vi "DAQmx_ControlLoop.vi"(8 "error in":errorcluster, 10 "DAQmx Task Name":refnum<k21>="MyVoltageTask_0", 11 "queue out":refnum<queue>) -> (0 "error out":errorcluster)   [LabVIEW 2013]
uses:
  DAQmx_Status.ctl
  <vilib>/Utility/error.llb/DialogType.ctl
  <vilib>/DAQmx/read.llb/DAQmx Read.vi
  <vilib>/DAQmx/read.llb/DAQmx Read (Analog 2D DBL NChan NSamp).vi
  <vilib>/Analysis/baseanly.llb/Mean (DBL).vi
  <vilib>/DAQmx/miscellaneous.llb/DAQmx Fill In Error Info.vi
  ControlDef/MiscParams.vi
  <vilib>/Analysis/NI_AALBase.lvlib
  <userlib>/Utility/ErrorLog_lib.lvlib
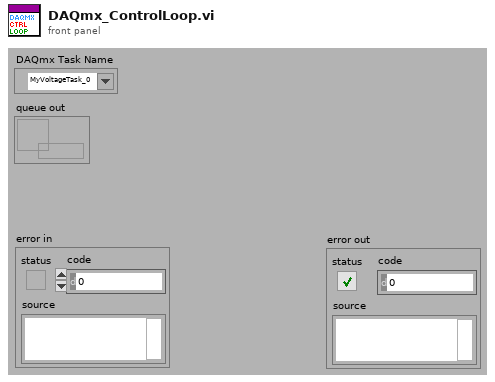
[diagram p1: front panel]
types:
  T1 = typedef "DAQmx_Status.ctl" = cluster{"State":enum16{"Initialize", "Idle", "Update", "Close", "Quit"}, "Para.":variant}
  T2 = enum16{"Initialize", "Idle", "Update", "Close", "Quit"}
  T3 = typedef "DialogType.ctl" = u16
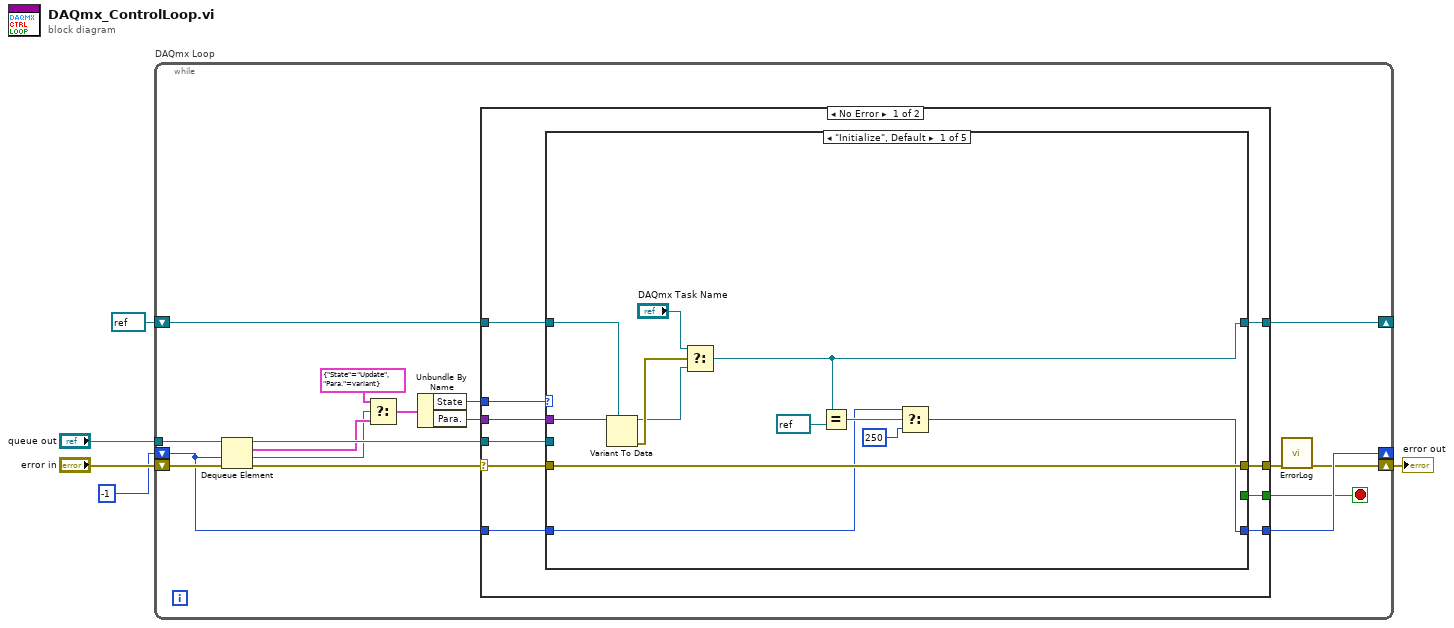
[diagram p0: block diagram]
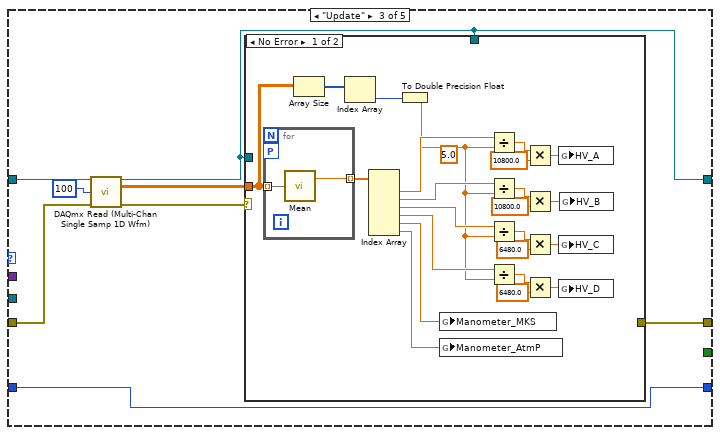
[diagram p3: hidden frame]
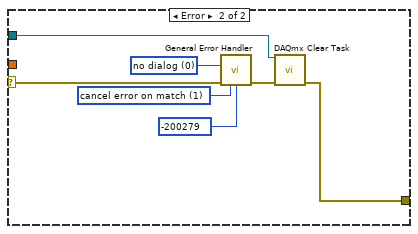
[diagram p4: hidden frame]
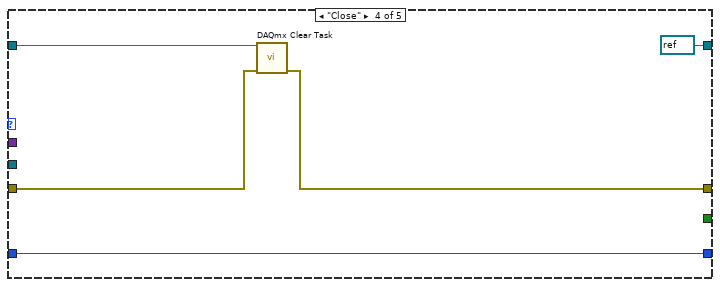
[diagram p5: hidden frame]
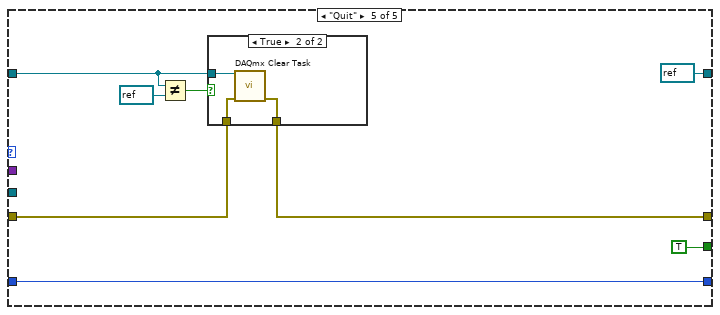
[diagram p6: hidden frame]
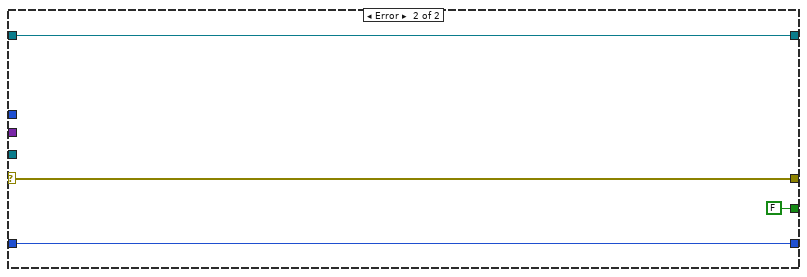
[diagram p8: hidden frame]
diagram:
  n1 = while "DAQmx Loop" {
    tunnel: "queue out" -> [w22]
    shift-right: [w7] -> w2
    shift-left: "error in" -> [w13]
    shift-right: [w11] -> _
    shift-left: refnum<k21> refnum ("DAQmx Task Name") -> [w10]
    shift-right: [w8] -> _
    shift-left: -1 -> [w9]
    stop <- w6 stop-if-true
    n2 = Dequeue Element(queue=w22, timeout in ms (-1)=w9, error in (no error)=w13) -> (queue out=w20:refnum<queue>, element=w17:T1, timed out?=w15:bool, error out=w19:errorcluster)
    n3 = Select(t=T1 {"State"=enum."Update", "Para."=variant}, s=w15, f=w17) -> (s? t:f=w18:T1)
    n4 = Unbundle By Name(w18) -> ("State"=w16:T2, "Para."=w21:variant)
    n5 = case shown="No Error" w19 {
      selector: w19 -> [w29 w108]
      tunnel: w16 -> [w32 _]
      tunnel: w21 -> [w24 _]
      tunnel: w20 -> [w27 _]
      tunnel: [w28 w108] -> w12
      tunnel: [w31 w107] -> w11
      tunnel: w10 -> [w30 w107]
      tunnel: w9 -> [w26 w106]
      tunnel: [w25 w106] -> w8
      tunnel: [w23 FALSE] -> w6
      frame No Error {
        n6 = case shown="\"Initialize\", Default" w32 {
          tunnel: [w37 w47 w49 refnum<k21> refnum ("DAQmx Task Name") refnum<k21> refnum ("DAQmx Task Name")] -> w31
          tunnel: w30 -> [w42 w47 w55 w92 w95]
          tunnel: w29 -> [w44 w46 w54 w91 w99]
          tunnel: [w44 w46 w50 w90 w98] -> w28
          tunnel: w27 -> [_ _ _ _ _]
          tunnel: w26 -> [w34 w45 w48 w88 w94]
          tunnel: [w35 w45 w48 w88 w94] -> w25
          tunnel: w24 -> [w43 _ _ _ _]
          tunnel: [_ _ _ _ TRUE] -> w23
          frame "Initialize", Default {
            n7 = Variant To Data(type=w42, Variant=w43) -> (data=w40:refnum<k21>, error out=w41:errorcluster)  [unwired: 1 in]
            n8 = Select(t="DAQmx Task Name", s=w41, f=w40) -> (s? t:f=w37:refnum<k21>)
            n9 = Equal?(x=w37, y=refnum<k21> refnum ("DAQmx Task Name")) -> (x = y?=w36:bool)
            n10 = Select(t=w34, s=w36, f=250) -> (s? t:f=w35:i32)
          }
          frame "Idle" {
          }
          frame "Update" {
            n11 = call-poly "DAQmx Read (Multi-Chan Single Samp 1D Wfm).vi"("task/channels in"=w55, "number of samples per channel"=100, "error in"=w54) -> ("task out"=w49:refnum<k21>, "data"=w52:dbl[][], "error out"=w51:errorcluster)  [unwired: 10 in]
            n12 = case shown="No Error" w51 {
              selector: w51 -> [_ w87]
              tunnel: w52 -> [w59 _]
              tunnel: [_ w83] -> w50
              tunnel: w49 -> [_ w82]
              tunnel: w49 -> [_ _]
              frame No Error {
                (unwired) 5.0 ("y")
                n13 = for {
                  tunnel: w59 -> [w80] mode=indexing
                  tunnel: [w79] -> w66 mode=indexing
                  workers-P: _ -> [_]
                  n14 = call-poly <vilib>:"Mean.vi"("X"=w80) -> ("mean"=w79:dbl)  [unwired: 1 out]
                }
                n15 = Array Size(array=w59) -> (size(s)=w58:i32[])
                n16 = Index Array(array=w58) -> (element=w57:i32)  [unwired: 1 in]
                n17 = Index Array(array=w66) -> (element #1=w65:dbl, element #2=w64:dbl, element #3=w63:dbl, element #4=w62:dbl, element #5=w61:dbl, element #6=w60:dbl)  [unwired: 6 in]
                n18 = To Double Precision Float(number=w57) -> (double precision float=w56:dbl)
                n19 = global write "MiscParams.vi" "Manometer_MKS"(w61) -> ()
                n20 = global write "MiscParams.vi" "Manometer_AtmP"(w60) -> ()
                n21 = Divide(x=w65, y=w56) -> (x/y=w78:dbl)
                n22 = Divide(x=w64, y=w56) -> (x/y=w75:dbl)
                n23 = Divide(x=w63, y=w56) -> (x/y=w71:dbl)
                n24 = Divide(x=w62, y=w56) -> (x/y=w72:dbl)
                n25 = Multiply(x=w78, y=10800.0) -> (x*y=w70:dbl)
                n26 = Multiply(x=w75, y=10800.0) -> (x*y=w69:dbl)
                n27 = Multiply(x=w71, y=6480.0) -> (x*y=w68:dbl)
                n28 = Multiply(x=w72, y=6480.0) -> (x*y=w67:dbl)
                n29 = global write "MiscParams.vi" "HV_A"(w70) -> ()
                n30 = global write "MiscParams.vi" "HV_C"(w68) -> ()
                n31 = global write "MiscParams.vi" "HV_D"(w67) -> ()
                n32 = global write "MiscParams.vi" "HV_B"(w69) -> ()
              }
              frame Error {
                w81 = T3 0 items=["no dialog", "OK message", "continue or stop message", "OK message + warnings", "continue/stop + warnings"] ("type of dialog (OK msg:1)")
                w86 = 1 items=["no exception", "cancel error on match", "set error on match"] ("[exception action] (none:0)")
                n33 = call <vilib>:"General Error Handler.vi"("type of dialog (OK msg:1)"=w81, "error in (no error)"=w87, "[exception action] (none:0)"=w86, "[exception code]"=-200279) -> ("error out"=w84:errorcluster)  [unwired: 7 in, 4 out]
                n34 = call <vilib>:"DAQmx Clear Task.vi"("task in"=w82, "error in"=w84) -> ("error out"=w83:errorcluster)  [unwired: 13 in]
              }
            }
          }
          frame "Close" {
            n35 = call <vilib>:"DAQmx Clear Task.vi"("task in"=w92, "error in"=w91) -> ("error out"=w90:errorcluster)  [unwired: 13 in]
          }
          frame "Quit" {
            n36 = Not Equal?(x=w95, y=refnum<k21> refnum ("DAQmx Task Name")) -> (x != y?=w96:bool)
            n37 = case shown="True" w96 {
              tunnel: w99 -> [w101 w104]
              tunnel: [w101 w103] -> w98
              tunnel: w95 -> [_ w102]
              frame False {
              }
              frame True {
                n38 = call <vilib>:"DAQmx Clear Task.vi"("task in"=w102, "error in"=w104) -> ("error out"=w103:errorcluster)  [unwired: 13 in]
              }
            }
          }
        }
      }
      frame Error {
      }
    }
    n39 = call <userlib>:"ErrorLog.vi"("error in (no error)"=w12) -> ("error out"=w7:errorcluster)  [unwired: 10 in]
  }
  "error out" <- w2
